vi "test_EnumsDatatype.vi"() -> ()   [LabVIEW 2013]
uses:
  source/TypeDescriptor/OpenDescriptor.lvlib
panel:
  out "Type":u8 format="%.0x"
  out "error out":errorcluster
  out "Default":variant
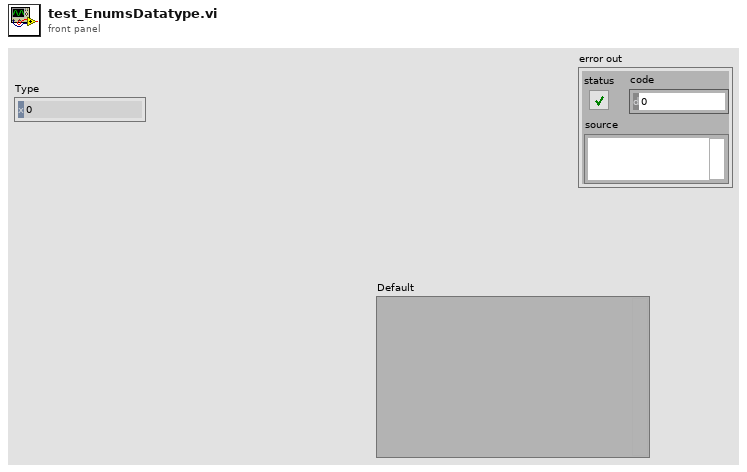
[diagram p1: front panel]
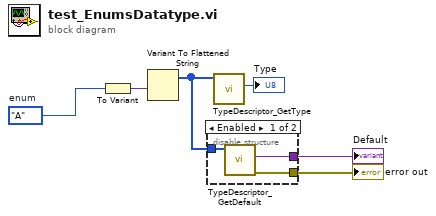
[diagram p0: block diagram]
diagram:
  w3 = enum16{"A", "B", "C"}."A"  # enum
  n1 = To Variant(anything=w3) -> (Variant=w4:variant)
  n2 = Variant To Flattened String(Variant=w4) -> (1:w1:i16[])  [unwired: 1 out]
  n3 = disable-structure shown="Enabled" {
    disable-tunnel: w1 -> [w9 _]
    disable-tunnel: [w8 _] -> w6
    disable-tunnel: [w7 _] -> w5
    frame Enabled {
      n4 = call "TypeDescriptor_GetDefault.vi"("type descriptor"=w9) -> ("error out"=w7:errorcluster, "Default"=w8:variant)  [unwired: 8 in, 1 out]
    }
    frame Disabled {
    }
  }
  "Default" <- w6
  "error out" <- w5
  n5 = call "TypeDescriptor_GetType.vi"("type descriptor"=w1) -> ("Type"=→"Type":u8)  [unwired: 9 in, 1 out]
